vi "RememberTargetLocation.vi"(11 "Target Data":T2) -> (3 "Peg Data":T1)   [LabVIEW 2016]
doc: "Combines encoder and gyro data to determine angle and distance to target even when target is not visible."
uses:
  Robot Global Data.vi
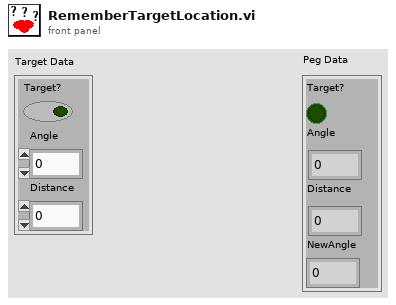
[diagram p1: front panel]
types:
  T1 = cluster{"Target?":bool, "Angle":dbl, "Distance":dbl, "NewAngle":dbl}
  T2 = cluster{"Target?":bool, "Angle":dbl, "Distance":dbl}
  T3 = cluster{bool, "Smallest B to A":dbl, "Distance":dbl, "Smallest B to A":dbl}
  T4 = cluster{"theta":dbl, "distance":dbl, "x":dbl, "y":dbl}[]
  T5 = cluster{"theta":dbl, "distance":dbl, "x":dbl, "y":dbl}
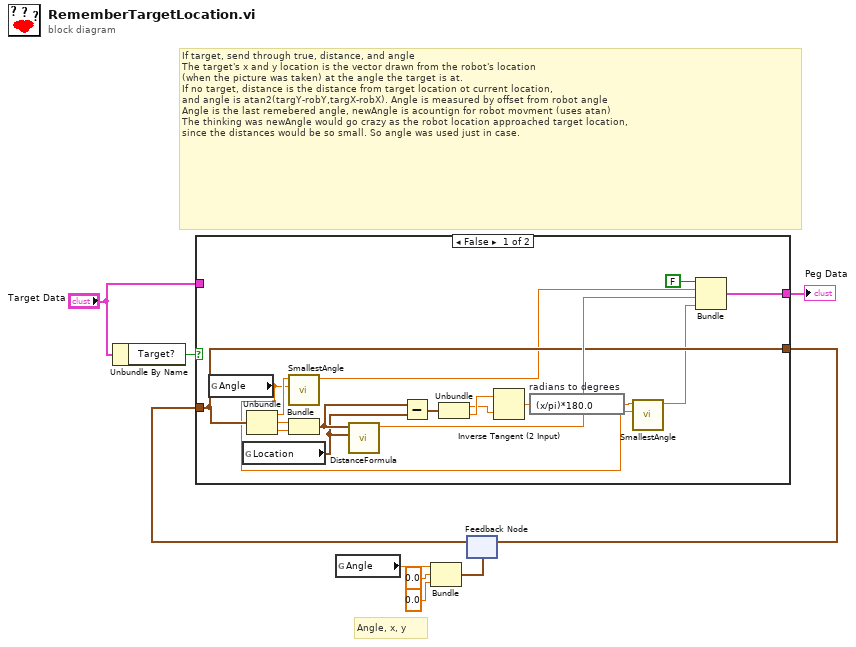
[diagram p0: block diagram]
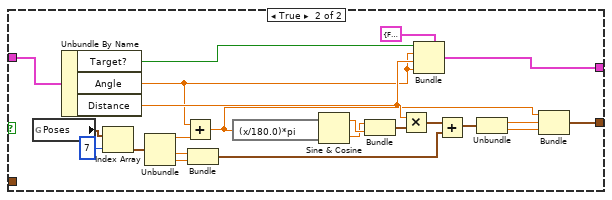
[diagram p2: hidden frame]
diagram:
  # "If target, send through true, distance, and angle\nThe target's x and y location is the vector drawn from the robot's location \n(when the picture was taken) at the angle the target is at. \nIf no target, distance is the distance from target location ot current location,\nand angle is atan2(targY-robY,targX-robX). Angle is measured by offset from robot angle\nAngle is the last remebered angle, newAngle is acountign for robot movment (uses atan)\nThe thinking was newAngle would go crazy as the robot location approached target location,\nsince the distances would be so small. So angle was used just in case."
  # "Angle, x, y"
  n1 = Unbundle By Name("Target Data") -> ("Target?"=w9:bool)
  n2 = global read "Robot Global Data.vi" "Angle"() -> (w7:dbl)
  n3 = Bundle("Angle"=w7, "Angle"=0.0, "Angle"=0.0) -> (w4:cluster{"Angle":dbl, "Angle":dbl, "Angle":dbl})  [unwired: 1 in]
  n4 = feedback #1(w4) -> (w3:cluster{"Angle":dbl, "Angle":dbl, "Angle":dbl})
  n5 = case shown="False" w9 {
    tunnel: "Target Data" -> [_ w33]
    tunnel: [w23 w32] -> w1
    tunnel: w3 -> [w20 _]
    tunnel: [w20 w34] -> w2
    frame False {
      n6 = global read "Robot Global Data.vi" "Angle"() -> (w10:dbl)
      n7 = global read "Robot Global Data.vi" "Location"() -> (w18:cluster{"x":dbl, "y":dbl})
      n8 = Unbundle(w20) -> ("Angle"=w24:dbl, "Angle"=w26:dbl, "Angle"=w25:dbl)
      n9 = call "SmallestAngle.vi"("Angle B"=w10, "Angle A"=w24) -> ("Smallest B to A"=w14:dbl)  [unwired: 9 in]
      n10 = Bundle("Angle"=w26, "Angle"=w25) -> (w19:cluster{"Angle":dbl, "Angle":dbl})  [unwired: 1 in]
      n11 = call "DistanceFormula.vi"("Point 2"=w18, "Point 1"=w19) -> ("Distance"=w21:dbl)  [unwired: 9 in]
      n12 = Subtract(x=w19, y=w18) -> (x-y=w17:cluster{dbl, dbl})
      n13 = Unbundle(w17) -> (w15:dbl, w16:dbl)
      n14 = Inverse Tangent (2 Input)(1:w15, 2:w16) -> (0:w13:dbl)
      n15 = expression code="(x/pi)*180.0" "radians to degrees"(w13) -> (w12:dbl)
      n16 = call "SmallestAngle.vi"("Angle B"=w10, "Angle A"=w12) -> ("Smallest B to A"=w11:dbl)  [unwired: 9 in]
      n17 = Bundle(FALSE, "Smallest B to A"=w14, "Distance"=w21, "Smallest B to A"=w11) -> (w23:T3)  [unwired: 1 in]
    }
    frame True {
      n18 = global read "Robot Global Data.vi" "Poses"() -> (w49:T4)
      n19 = Unbundle By Name(w33) -> ("Target?"=w30:bool, "Angle"=w28:dbl, "Distance"=w29:dbl)
      n20 = Index Array(array=w49, index=7) -> (element=w47:T5)
      n21 = Unbundle(w47) -> ("theta"=w46:dbl, "x"=w40:dbl, "y"=w39:dbl)  [unwired: 1 out]
      n22 = Add(x=w28, y=w46) -> (x+y=w27:dbl)
      n23 = Bundle("x"=w40, "y"=w39) -> (w38:cluster{"x":dbl, "y":dbl})  [unwired: 1 in]
      n24 = expression code="(x/180.0)*pi" ("degrees to radians")(w27) -> (w45:dbl)
      n25 = Sine & Cosine(0:w45) -> (1:w44:dbl, 2:w43:dbl)
      n26 = Bundle(w43, w44) -> (w42:cluster{dbl, dbl})  [unwired: 1 in]
      n27 = Multiply(x=w29, y=w42) -> (x*y=w41:cluster{dbl, dbl})
      n28 = Bundle(cluster=T1 {"Target?"=FALSE, "Angle"=0.0, "Distance"=0.0, "NewAngle"=0.0} ("Peg Dat"), "Target?"=w30, "Angle"=w28, "Distance"=w29, "NewAngle"=w28) -> (w32:T1)
      n29 = Add(x=w41, y=w38) -> (x+y=w37:cluster{dbl, dbl})
      n30 = Unbundle(w37) -> (w36:dbl, w35:dbl)
      n31 = Bundle(w27, w36, w35) -> (w34:cluster{dbl, dbl, dbl})  [unwired: 1 in]
    }
  }
  "Peg Data" <- w1
  n32 = feedback-in #1(w2) -> ()
